vi "MIDI Parse Entry.vi"(6 "Error":bool=TRUE, 8 "Running State":string="-", 9 "Datastring":string, 10 "MIDI Tag":string="Databyte", 11 "MIDI Parse Data in":T1 {"Current Byte" format="%.0x"; "Running Statusbyte" format="%.0x"; "MIDI-Bytes In" format="%.0x"}) -> (3 "MIDI Parse Data out":T1 {"Current Byte" format="%.0x"; "Running Statusbyte" format="%.0x"; "MIDI-Bytes In" format="%.0x"})   [LabVIEW 2019]
uses:
  Controls/Parser-data.ctl
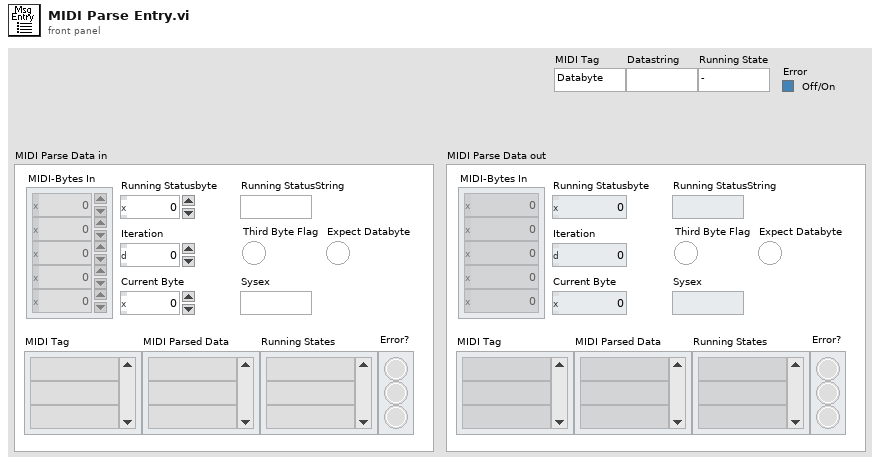
[diagram p1: front panel]
types:
  T1 = typedef "Parser-data.ctl" = cluster{"MIDI-Bytes In":u8[], "MIDI Tag":string[], "MIDI Parsed Data":string[], "Iteration":i32, "Error?":bool[], "Running States":string[], "Running Statusbyte":u8, "Running StatusString":string, "Third Byte Flag":bool, "Current Byte":u8, "Sysex":string, "Expect Databyte":bool}
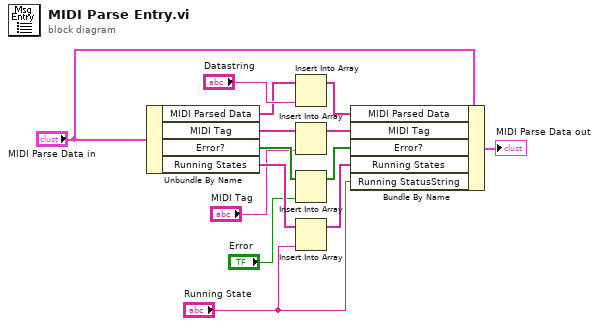
[diagram p0: block diagram]
diagram:
  n1 = Unbundle By Name("MIDI Parse Data in") -> ("MIDI Parsed Data"=w2:string[], "MIDI Tag"=w4:string[], "Error?"=w6:bool[], "Running States"=w8:string[])
  n2 = Insert Into Array(array=w2, new element="Datastring") -> (w10:string[])  [unwired: 1 in]
  n3 = Insert Into Array(array=w4, new element="MIDI Tag") -> (w11:string[])  [unwired: 1 in]
  n4 = Insert Into Array(array=w6, new element="Error") -> (w12:bool[])  [unwired: 1 in]
  n5 = Insert Into Array(array=w8, new element="Running State") -> (w13:string[])  [unwired: 1 in]
  n6 = Bundle By Name(cluster="MIDI Parse Data in", "MIDI Parsed Data"=w10, "MIDI Tag"=w11, "Error?"=w12, "Running States"=w13, "Running StatusString"="Running State") -> (→"MIDI Parse Data out":T1)
